vi "Create Child Instrument SMO.vi"(8 "error in (no error)":errorcluster) -> (0 "error out":errorcluster)   [LabVIEW 2016]
uses:
  lvsrc/SMOs/Example Instrument/Example Instrument.lvclass
  C:/Program Files (x86)/National Instruments/LabVIEW 2016/vi.lib/JKI/JKI SMO/SMO/SMO.lvclass
  <vilib>/JKI/JKI SMO/SMO/SMO.lvclass
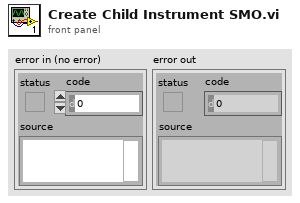
[diagram p1: front panel]
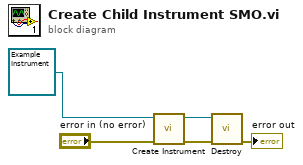
[diagram p0: block diagram]
diagram:
  n1 = call-dynamic "Create Instrument.vi"("error in (no error)"="error in (no error)", "Instrument in"=refnum<class "Example Instrument.lvclass"> refnum ("Example Instrument.lvclass")) -> ("error out"=w4:errorcluster, "Instrument out"=w3:refnum<class "Example Instrument.lvclass">)  [unwired: 8 in]
  n2 = call <vilib>:"Destroy.vi"("error in (no error)"=w4, "SMO"=w3) -> ("error out"=→"error out":errorcluster)  [unwired: 9 in]
